vi "Open-Close-Relays-Arduino.vi"(8 "error In":errorcluster, 11 "Select Com Port":refnum<visa-resource-name>) -> (0 "error Out":errorcluster, 2 "Output String":string, 3 "return count":u32)   [LabVIEW 2020]
uses:
  select-Action.ctl
  <vilib>/Instr/_visa.llb/VISA Set IO Buffer Mask.ctl
  <vilib>/Instr/_visa.llb/VISA Configure Serial Port (Instr).vi
panel:
  in  "Select Action":T1
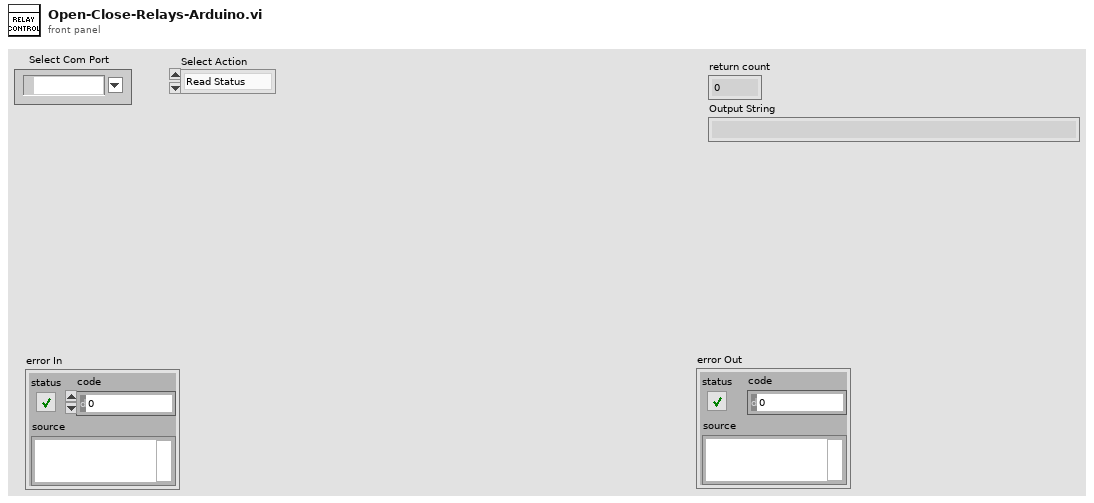
[diagram p1: front panel]
types:
  T1 = typedef "select-Action.ctl" = enum16{"Read Status", "Open Relays", "Close Relays", "Reset"}
  T2 = enum16{"Native", "Native Command Line", "UNIX", "Macintosh", "DOS"}
  T3 = typedef "VISA Set IO Buffer Mask.ctl" = u16
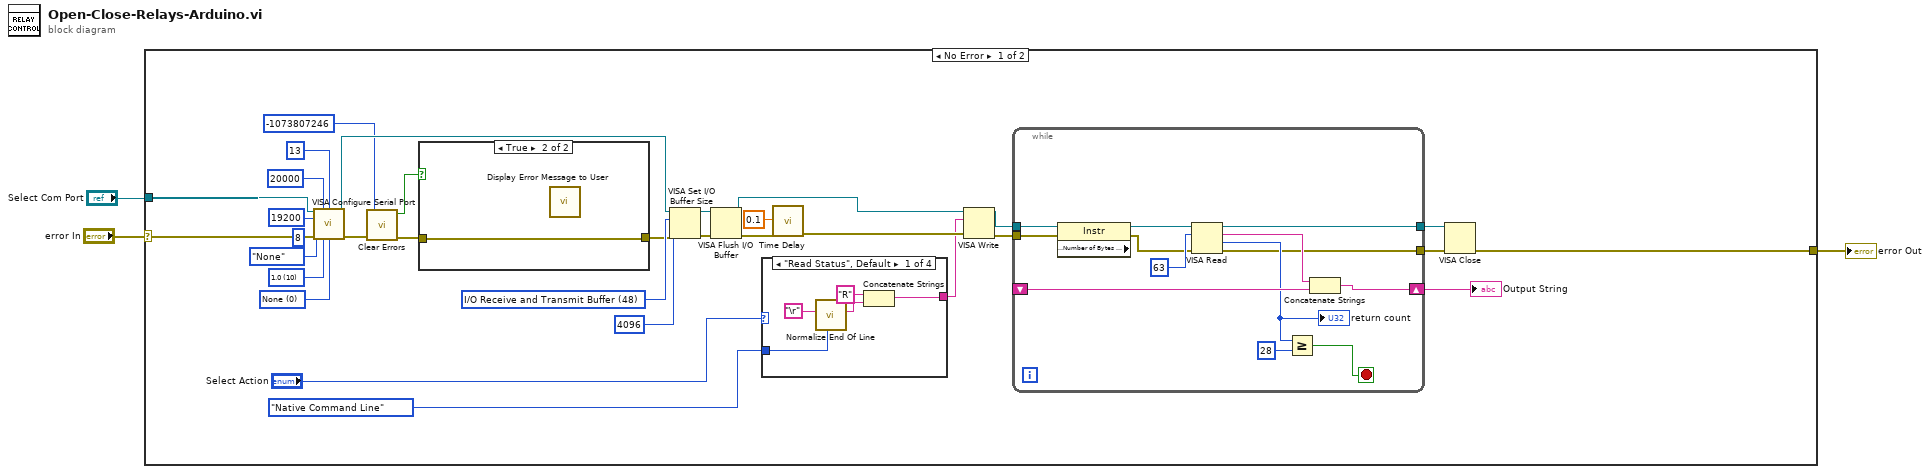
[diagram p0: block diagram]
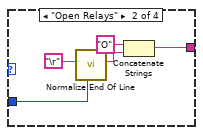
[diagram p2: hidden frame]
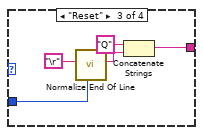
[diagram p3: hidden frame]
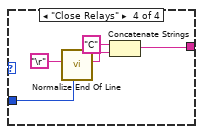
[diagram p4: hidden frame]
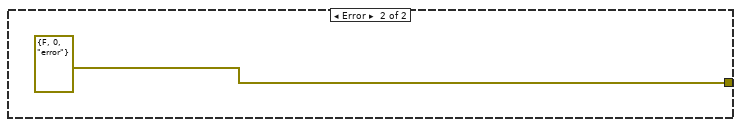
[diagram p6: hidden frame]
diagram:
  n1 = case shown="No Error" "error In" {
    selector: "error In" -> [w35 _]
    tunnel: [w14 errorcluster {"status"=FALSE, "code"=0, "source"="error"} ("error IO")] -> w2
    tunnel: "Select Com Port" -> [w34 _]
    frame No Error {
      w25 = T3 48 items=["I/O Receive Buffer"=16, "I/O Transmit Buffer"=32, "I/O Receive and Transmit Buffer"=48] ("Mask")
      w29 = u16 0 items=["None", "XON/XOFF", "RTS/CTS", "XON/XOFF & RTS/CTS", "DTR/DSR", "XON/XOFF & DTR/DSR"] ("flow control (0:none)")
      w30 = u16 10 items=["1.0"=10, "1.5"=15, "2.0"=20] ("stop bits (10: 1 bit)")
      n2 = call-poly "VISA Configure Serial Port"("VISA resource name"=w34, "timeout (10sec)"=u32 20000, "termination char\n(0xA = '\\n' = LF)"=u8 13 ("termination char\n(0xA = '\\n' = LF)"), "baud rate (9600)"=u32 19200, "data bits (8)"=u16 8, "parity (0:none)"=enum16{"None", "Odd", "Even", "Mark", "Space"}."None", "error in (no error)"=w35, "stop bits (10: 1 bit)"=w30, "flow control (0:none)"=w29) -> ("VISA resource name out"=w28:refnum<visa-resource-name>, "error out"=w8:errorcluster)  [unwired: 5 in]
      n3 = call <vilib>:"Clear Errors.vi"("error in (no error)"=w8, "specific error code to clear (0: all)"=-1073807246) -> ("error out"=w7:errorcluster, "specific error cleared?"=w6:bool)  [unwired: 4 in]
      n4 = case shown="True" w6 {
        tunnel: [w56 w57] -> w10
        tunnel: w7 -> [w56 w57]
        frame False {
        }
        frame True {
          n5 = call "Display Error Message to User"() -> ()  [unwired: 10 in, 2 out]
        }
      }
      n6 = VISA Set I/O Buffer Size(VISA resource name=w28, mask (16)=w25, size (4096)=u32 4096, error in (no error)=w10) -> (VISA resource name out=w26:refnum<visa-resource-name>, error out=w27:errorcluster)
      n7 = VISA Flush I/O Buffer(VISA resource name=w26, error in (no error)=w27) -> (VISA resource name out=w22:refnum<visa-resource-name>, error out=w23:errorcluster)  [unwired: 1 in]
      n8 = case shown="\"Read Status\", Default" "Select Action" {
        tunnel: T2."Native Command Line" ("end of line (Native)") -> [w36 w43 w48 w51]
        tunnel: [w37 w41 w46 w52] -> w19
        frame "Read Status", Default {
          n9 = call <vilib>:"Normalize End Of Line.vi"("end of line (Native)"=w36, "string in"="\r") -> ("string out"=w40:string)  [unwired: 6 in]
          n10 = Concatenate Strings("R" ("string"), w40) -> (w37:string)
        }
        frame "Open Relays" {
          n11 = call <vilib>:"Normalize End Of Line.vi"("end of line (Native)"=w43, "string in"="\r") -> ("string out"=w45:string)  [unwired: 6 in]
          n12 = Concatenate Strings("O" ("string"), w45) -> (w41:string)
        }
        frame "Reset" {
          n13 = call <vilib>:"Normalize End Of Line.vi"("end of line (Native)"=w48, "string in"="\r") -> ("string out"=w50:string)  [unwired: 6 in]
          n14 = Concatenate Strings("Q" ("string"), w50) -> (w46:string)
        }
        frame "Close Relays" {
          n15 = call <vilib>:"Normalize End Of Line.vi"("end of line (Native)"=w51, "string in"="\r") -> ("string out"=w55:string)  [unwired: 6 in]
          n16 = Concatenate Strings("C" ("string"), w55) -> (w52:string)
        }
      }
      n17 = call "Time Delay"("error in (no error)"=w23, "Delay Time (s)"=0.1) -> ("error out"=w21:errorcluster)  [unwired: 9 in]
      n18 = VISA Write(VISA resource name=w22, write buffer=w19, error in (no error)=w21) -> (VISA resource name out=w17:refnum<visa-resource-name>, error out=w18:errorcluster)  [unwired: 1 out]
      n19 = while {
        tunnel: w18 -> [w70]
        tunnel: w17 -> [w69]
        shift-right: [w61] -> w5
        shift-left: _ -> [w62]
        tunnel: [w59] -> w16
        tunnel: [w58] -> w15
        stop <- w65 stop-if-true
        n20 = property class="Instr" props=["Serial Settings:Number of Bytes at Serial Port"](reference=w69, error in=w70) -> (reference out=w68:refnum<visa-resource-name>, error out=w66:errorcluster)  [unwired: 1 out]
        n21 = VISA Read(VISA resource name=w68, byte count=u32 63, error in (no error)=w66) -> (VISA resource name out=w59:refnum<visa-resource-name>, read buffer=w63:string, return count=w60:u32, error out=w58:errorcluster)
        "return count" <- w60
        n22 = Greater Or Equal?(x=w60, y=u32 28) -> (x >= y?=w65:bool)
        n23 = Concatenate Strings(w63, w62) -> (w61:string)
      }
      "Output String" <- w5
      n24 = VISA Close(VISA resource name=w16, error in (no error)=w15) -> (error out=w14:errorcluster)
    }
    frame Error {
    }
  }
  "error Out" <- w2
